vi "Write image path.vi"(8 "error in (no error)":errorcluster, 10 "image path":path, 11 "data_loder_single_image in":refnum<class "data_loder_single_image.lvclass">) -> (0 "error out":errorcluster, 3 "data_loder_single_image out":refnum<class "data_loder_single_image.lvclass">)   [LabVIEW 2017, in "data_loder_single_image.lvclass"]
uses:
  data_loder_single_image.lvclass
  data_loder_single_image.lvclass/data_loder_single_image.ctl
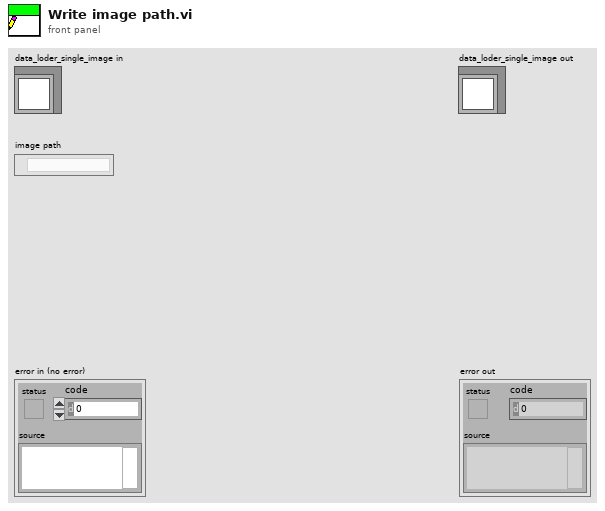
[diagram p1: front panel]
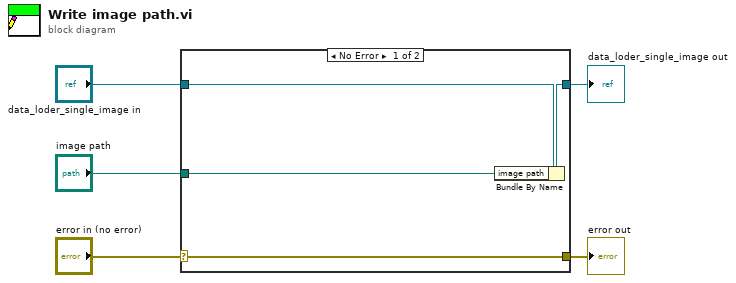
[diagram p0: block diagram]
diagram:
  n1 = case shown="No Error" "error in (no error)" {
    selector: "error in (no error)" -> [w9 w10]
    tunnel: [w9 w10] -> w4
    tunnel: [w7 w11] -> w2
    tunnel: "data_loder_single_image in" -> [w8 w11]
    tunnel: "image path" -> [w6 _]
    frame No Error {
      n2 = Bundle By Name(cluster=w8, "image path"=w6) -> (w7:refnum<class "data_loder_single_image.lvclass">)
    }
    frame Error {
    }
  }
  "error out" <- w4
  "data_loder_single_image out" <- w2
